vi "Stop Core.vi"(10 "final error code":i32, 11 "ConfigurableActor in":refnum<class "ConfigurableActor.lvclass">) -> (3 "ConfigurableActor out":refnum<class "ConfigurableActor.lvclass">)   [LabVIEW 2014, in "ConfigurableActor.lvclass"]
doc: "(<B>Filename</B>: Actor Framework.lvlib:Actor.lvclass:Stop Core.vi)\n\nDefines what the actor does before it stops. Use the <B>final error code</B> input to determine whether the actor shut down in response to an error.\n\nBy default, this method does nothing. A descendant class may override it to define behavior, such as shutting down any processes the actor initiated in its override of the Actor Core method."
uses:
  ConfigurableActor.lvclass
  ConfigurableActor.lvclass/ConfigurableActor.ctl
  <vilib>/ActorFramework/Actor/Actor.lvclass
  <vilib>/LabVIEW Open Source/Configuration Manager/Manager/ConfigManager.lvclass
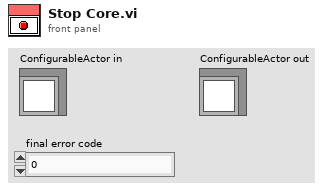
[diagram p1: front panel]
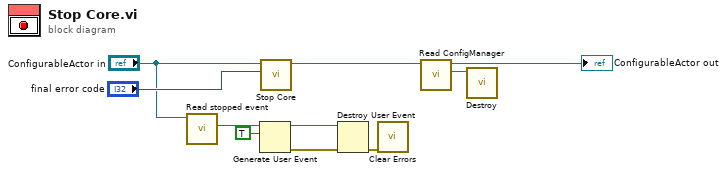
[diagram p0: block diagram]
diagram:
  n1 = call "Read stopped event.vi"("ConfigurableActor in"="ConfigurableActor in") -> ("stopped event"=w8:refnum<user-event>)  [unwired: 8 in, 2 out]
  n2 = Generate User Event(user event=w8, event data cluster=TRUE ("event data")) -> (user event out=w6:refnum<user-event>, error out=w5:errorcluster)  [unwired: 2 in]
  n3 = call-parent "Stop Core.vi"("final error code"="final error code", "Actor in"="ConfigurableActor in") -> ("Actor out"=w3:refnum<class "ConfigurableActor.lvclass">)  [unwired: 9 in]
  n4 = Destroy User Event(user event=w6, error in=w5) -> (error out=w4:errorcluster)
  n5 = call <vilib>:"Clear Errors.vi"("error in (no error)"=w4) -> ()  [unwired: 5 in, 2 out]
  n6 = call "Read ConfigManager.vi"("ConfigurableActor in"=w3) -> ("ConfigManager"=w1:refnum<class "ConfigManager.lvclass">, "ConfigurableActor out"=→"ConfigurableActor out":refnum<class "ConfigurableActor.lvclass">)  [unwired: 8 in, 1 out]
  n7 = call-dynamic "Destroy.vi"("ConfigManager in"=w1) -> ()  [unwired: 9 in, 2 out]
